vi "ex_Match String with Wildcards.vi"(10 "Signal Name With Wildcards":string, 11 "Signal Name to Test":string) -> (0 "offset past match":i32, 2 "match substring":string, 3 "x = y?":bool)   [LabVIEW 2020]
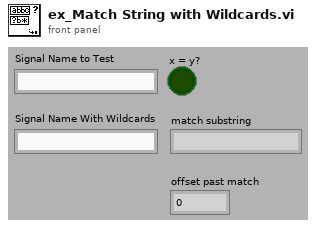
[diagram p1: front panel]
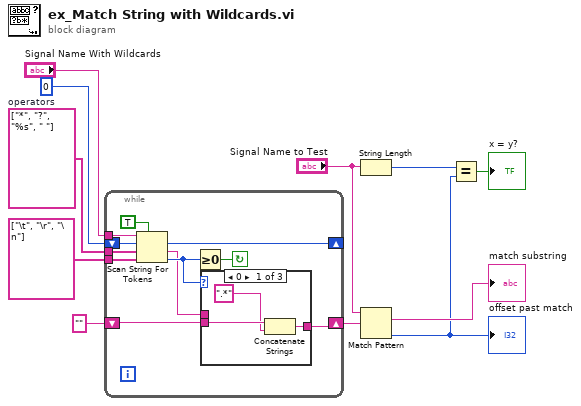
[diagram p0: block diagram]
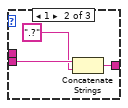
[diagram p2: hidden frame]
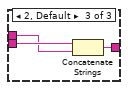
[diagram p3: hidden frame]
diagram:
  w11 = string[] ["*", "?", "%s", " "]  # operators
  n1 = while {
    tunnel: w11 -> [w22]
    shift-right: [w21] -> _
    shift-left: 0 ("offset past token") -> [w20]
    tunnel: "Signal Name With Wildcards" -> [w18]
    tunnel: string[] ["\t", "\r", "\n"] ("delimiters (\\s,\\t,\\r,\\n)") -> [w16]
    shift-right: [w12] -> w7
    shift-left: "" -> [w13]
    stop <- w19 continue-if-true
    n2 = Scan String For Tokens(5:TRUE ("allow empty tokens? (F)"), 6:w16, 7:w22, 8:w20, 9:w18) -> (0:w15:i32, 1:w14:string, 2:w21:i32)  [unwired: 1 in, 1 out]
    n3 = Greater Or Equal To 0?(x=w15) -> (x >= 0?=w19:bool)
    n4 = case shown="0" w15 {
      tunnel: w14 -> [_ _ w30]
      tunnel: w13 -> [w25 w27 w31]
      tunnel: [w24 w28 w29] -> w12
      frame 0 {
        n5 = Concatenate Strings(w25, ".*") -> (w24:string)
      }
      frame 1 {
        n6 = Concatenate Strings(w27, ".?") -> (w28:string)
      }
      frame 2, Default {
        n7 = Concatenate Strings(w31, w30) -> (w29:string)
      }
    }
  }
  n8 = String Length(string="Signal Name to Test") -> (length=w4:i32)
  n9 = Match Pattern(string="Signal Name to Test", regular expression=w7) -> (match substring=→"match substring":string, offset past match=w3:i32)  [unwired: 1 in, 2 out]
  "offset past match" <- w3
  n10 = Equal?(x=w4, y=w3) -> (x = y?=→"x = y?":bool)
